vi "Wave2D_Cal UPT.vi"(10 "P":T2, 11 "U":dbl[][](array[numeric])) -> (0 "error":i32, 3 "UPT":dbl[][](array[numeric]))   [LabVIEW 2017, in "NI_PDE.lvlib"]
uses:
  <vilib>/gmath/NI_PDE.lvlib
  <vilib>/Analysis/Matrix/Datatypes/RealMatrix.ctl
  <vilib>/Analysis/baseanly.llb/Real A x B.vi
  <vilib>/Analysis/NI_AALBase.lvlib
  <vilib>/Analysis/Matrix/NI_Matrix.lvlib
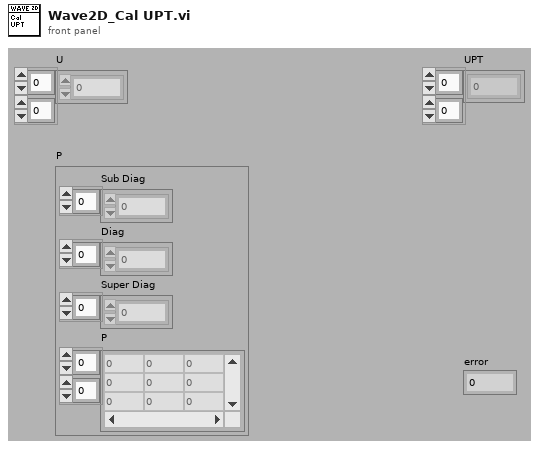
[diagram p1: front panel]
types:
  T1 = typedef "NI_Matrix.lvlib/RealMatrix.ctl" = dbl[][]
  T2 = cluster{"Sub Diag":dbl[], "Diag":dbl[], "Super Diag":dbl[], "P":T1}
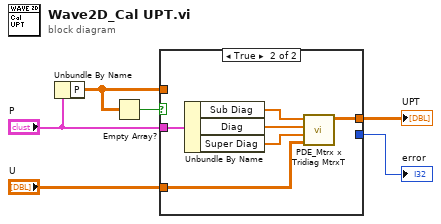
[diagram p0: block diagram]
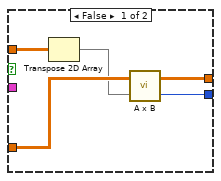
[diagram p2: hidden frame]
diagram:
  n1 = Unbundle By Name("P") -> ("P"=w4:T1)
  n2 = Empty Array?(array=w4) -> (empty?=w6:bool)
  n3 = case shown="True" w6 {
    tunnel: "U" -> [w9 w13]
    tunnel: w4 -> [w8 _]
    tunnel: [w11 w12] -> w3
    tunnel: [w10 _] -> w1
    tunnel: "P" -> [_ w17]
    frame False {
      n4 = Transpose 2D Array(2D array=w8) -> (transposed array=w7:T1)
      n5 = call-poly <vilib>:"A x B.vi"("B"=w7, "A"=w9) -> ("error"=w10:i32, "A x B"=w11:T1)
    }
    frame True {
      n6 = Unbundle By Name(w17) -> ("Sub Diag"=w16:dbl[], "Diag"=w15:dbl[], "Super Diag"=w14:dbl[])
      n7 = call <vilib>:"PDE_Mtrx x Tridiag MtrxT.vi"("X"=w13, "Super Diag"=w14, "Diag"=w15, "Sub Diag"=w16) -> ("X x MtrxT"=w12:dbl[][])  [unwired: 7 out]
    }
  }
  "UPT" <- w3
  "error" <- w1
